vi "Configure Measurement (Phase Noise).vi"(0 "VISA resource name":refnum<visa-resource-name>, 1 "Spurious Mode (0: Normalized)":u16(ring) items=["Normalized (dBc/Hz)", "Power (dBc)", "Omit"], 5 "Intermediate Frequency Gain (20 dB)":i32=20 format="%^#_9g", 7 "Correlation (1)":i32=1 format="%^#_9g", 9 "Local Bandwidth Optimization (1: Wide)":u16(ring)=1 items=["Narrow", "Wide"], 11 "error in (no error)":errorcluster, 12 "Minimum Spur Level (-500 dBc)":dbl=-500.0 format="%^#_9g") -> (4 "VISA resource name out":refnum<visa-resource-name>, 15 "error out":errorcluster)   [LabVIEW 2011, in "Agilent E5052X.lvlib"]
doc: "Configures the instrument to take Phase Noise measurements.\n\n<b>Note: </b>\n\n \"Configure Measurement Characteristics(Phase Noise)\" VI must be called before calling this VI."
uses:
  Agilent E5052X.lvlib
panel:
  # "Spurious Settings"
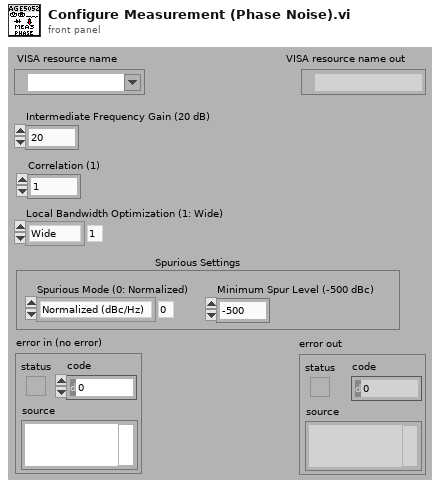
[diagram p1: front panel]
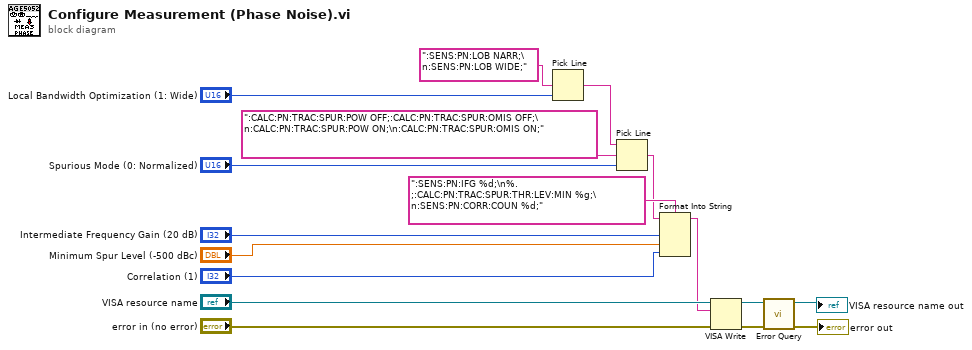
[diagram p0: block diagram]
diagram:
  n1 = Pick Line(multi-line string=":SENS:PN:LOB NARR;\n:SENS:PN:LOB WIDE;", line index="Local Bandwidth Optimization (1: Wide)") -> (output string=w3:string)  [unwired: 1 in]
  n2 = Pick Line(string ("")=w3, multi-line string=":CALC:PN:TRAC:SPUR:POW OFF;:CALC:PN:TRAC:SPUR:OMIS OFF;\n:CALC:PN:TRAC:SPUR:POW ON;\n:CALC:PN:TRAC:SPUR:OMIS ON;", line index="Spurious Mode (0: Normalized)") -> (output string=w2:string)
  n3 = Format Into String(format string=":SENS:PN:IFG %d;\n%.;:CALC:PN:TRAC:SPUR:THR:LEV:MIN %g;\n:SENS:PN:CORR:COUN %d;", initial string=w2, "Intermediate Frequency Gain (20 dB)", "Minimum Spur Level (-500 dBc)", "Correlation (1)") -> (resulting string=w1:string)  [unwired: 1 in, 1 out]
  n4 = VISA Write(VISA resource name="VISA resource name", write buffer=w1, error in (no error)="error in (no error)") -> (VISA resource name out=w12:refnum<visa-resource-name>, error out=w11:errorcluster)  [unwired: 1 out]
  n5 = call "Error Query.vi"("error in (no error)"=w11, "VISA resource name"=w12) -> ("error out"=→"error out":errorcluster, "VISA resource name out"=→"VISA resource name out":refnum<visa-resource-name>)  [unwired: 6 in, 2 out]
